vi "Initialize.vi"(0 "Universal Robot in":refnum<class "Universal Robot.lvclass">, 1 "DashboardServer":refnum<class "Dashboard Server.lvclass">, 5 "error in (no error)":errorcluster) -> (14 "Universal Robot out":refnum<class "Universal Robot.lvclass">, 19 "error out":errorcluster)   [LabVIEW 2016, in "Universal Robot.lvclass"]
uses:
  Universal Robot.lvclass
  DashboardServer/Dashboard Server.lvclass
  Universal Robot.lvclass/Universal Robot.ctl
  ProgramControlEvent.ctl
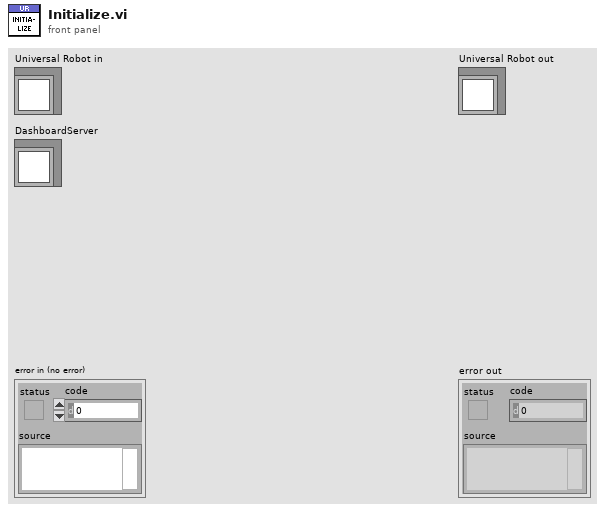
[diagram p1: front panel]
types:
  T1 = typedef "Universal Robot.lvclass/ProgramControlEvent.ctl" = enum16{"Stop", "Pause"}
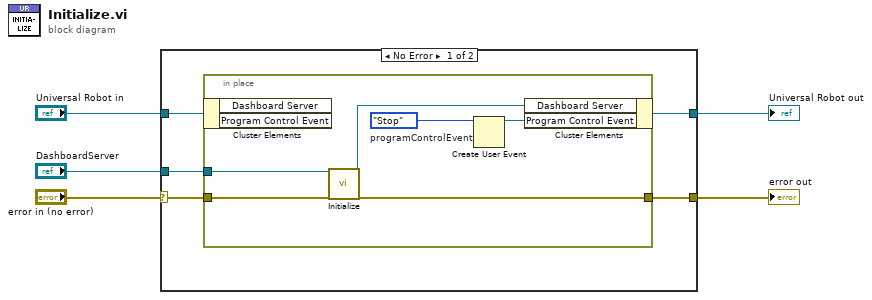
[diagram p0: block diagram]
diagram:
  n1 = case shown="No Error" "error in (no error)" {
    selector: "error in (no error)" -> [w10 w18]
    tunnel: [w8 w18] -> w4
    tunnel: [w6 w17] -> w2
    tunnel: "Universal Robot in" -> [w7 w17]
    tunnel: "DashboardServer" -> [w9 _]
    frame No Error {
      n2 = in-place {
        in-place-border: w10 -> [w16]
        in-place-border: w9 -> [w15]
        in-place-border: [w14] -> w8
        w11 = ProgramControlEvent."Stop"  # programControlEvent
        n3 = in-place-cluster #1(w7) -> ()  [unwired: 2 out]
        n4 = call-dynamic "Initialize.vi"("DashboardServer in"=w15, "error in (no error)"=w16) -> ("DashboardServer out"=w13:refnum<class "Dashboard Server.lvclass">, "error out"=w14:errorcluster)  [unwired: 16 in]
        n5 = Create User Event(user event datatype=w11) -> (user event=w12:refnum<user-event>)  [unwired: 1 in, 1 out]
        n6 = in-place-cluster #1("Dashboard Server"=w13, "Program Control Event"=w12) -> (w6:refnum<class "Universal Robot.lvclass">)
      }
    }
    frame Error {
    }
  }
  "error out" <- w4
  "Universal Robot out" <- w2
